vi "Read DEV INI.vi"(8 "Error In":errorcluster, 11 "Firmware INI Path":path) -> (0 "Error Out":errorcluster, 2 "Device Data":T1, 3 "Duplicate Firmware INI Path":path)   [LabVIEW 2011, in "LMH-LINX.lvlib"]
uses:
  LMH-LINX.lvlib
  Type Defs/Device Data.ctl
  <vilib>/Utility/config.llb/Read Key (String).vi
  <vilib>/Utility/config.llb/Read Key (I32).vi
  <vilib>/Utility/config.llb/NI_LVConfig.lvlib
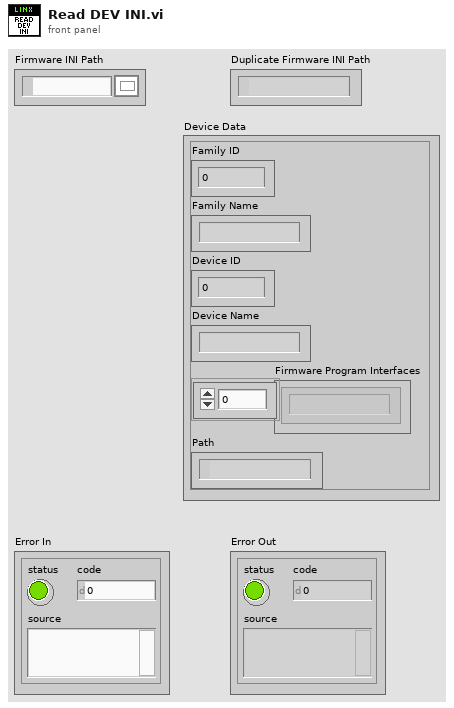
[diagram p1: front panel]
types:
  T1 = typedef "LMH-LINX.lvlib/Device Data.ctl" = cluster{"Family ID":i32, "Family Name":string, "Device ID":i32, "Device Name":string, "Firmware Program Interfaces":string[], "Path":path}
  T2 = typedef "NI_LVConfig.lvlib/Config Data RefNum.ctl" = refnum<k1>
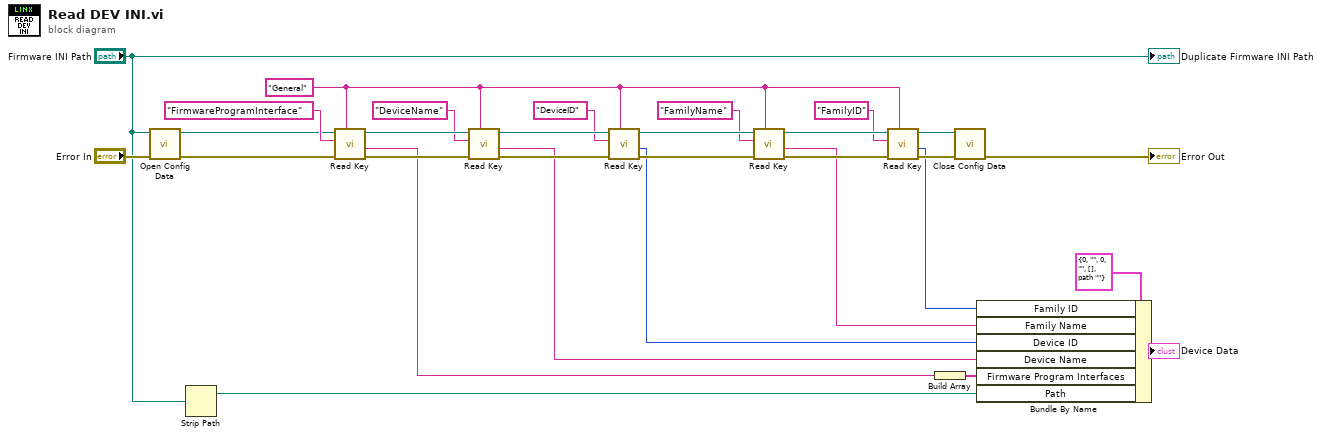
[diagram p0: block diagram]
diagram:
  w15 = "General" ("key")
  n1 = call <vilib>:"Open Config Data.vi"("error in (no error)"="Error In", "configuration file path"="Firmware INI Path") -> ("error out"=w29:errorcluster, "refnum"=w26:T2)  [unwired: 7 in, 1 out]
  n2 = Strip Path(path="Firmware INI Path") -> (stripped path=w3:path)  [unwired: 1 out]
  n3 = call-poly <vilib>:"Read Key.vi"("section"=w15, "error in (no error)"=w29, "key"="FirmwareProgramInterface", "refnum"=w26) -> ("error out"=w19:errorcluster, "value"=w1:string, "refnum out"=w20:T2)  [unwired: 4 in, 1 out]
  n4 = call-poly <vilib>:"Read Key.vi"("section"=w15, "error in (no error)"=w19, "key"="DeviceName", "refnum"=w20) -> ("error out"=w18:errorcluster, "value"=w6:string, "refnum out"=w21:T2)  [unwired: 4 in, 1 out]
  n5 = call-poly <vilib>:"Read Key.vi"("section"=w15, "error in (no error)"=w18, "key"="DeviceID", "refnum"=w21) -> ("error out"=w17:errorcluster, "value"=w7:i32, "refnum out"=w22:T2)  [unwired: 4 in, 1 out]
  n6 = call-poly <vilib>:"Read Key.vi"("section"=w15, "error in (no error)"=w17, "key"="FamilyName", "refnum"=w22) -> ("error out"=w16:errorcluster, "value"=w8:string, "refnum out"=w23:T2)  [unwired: 4 in, 1 out]
  n7 = call-poly <vilib>:"Read Key.vi"("section"=w15, "error in (no error)"=w16, "key"="FamilyID", "refnum"=w23) -> ("error out"=w25:errorcluster, "value"=w9:i32, "refnum out"=w24:T2)  [unwired: 4 in, 1 out]
  n8 = Build Array(w1) -> (w2:string[])
  n9 = call <vilib>:"Close Config Data.vi"("error in (no error)"=w25, "refnum"=w24) -> ("error out"=→"Error Out":errorcluster)  [unwired: 8 in, 1 out]
  n10 = Bundle By Name(cluster=T1 {"Family ID"=0, "Family Name"="", "Device ID"=0, "Device Name"="", "Firmware Program Interfaces"=[], "Path"=path ""} ("Device Data"), "Family ID"=w9, "Family Name"=w8, "Device ID"=w7, "Device Name"=w6, "Firmware Program Interfaces"=w2, "Path"=w3) -> (→"Device Data":T1)
  "Duplicate Firmware INI Path" <- "Firmware INI Path"
